vi "Example_SingleSquare.vi"() -> ()   [LabVIEW 2019, in "VGA.lvlib"]
doc: "Use this VI to test Monitor pixel-perfect. 0= top left pixel, 307199 = bottom right pixel."
uses:
  VGA.lvlib
  <vilib>/Platform/TimedLoop/XDataNode/timing_clust.ctl
  <vilib>/Platform/TimedLoop/XDataNode/nitl_modes.ctl
  <vilib>/Platform/TimedLoop/XDataNode/wakeup.ctl
  <vilib>/rvi/Emulation/niFpgaGetClockAttributes.vi
  <vilib>/rvi/Emulation/niFpgaSctlEmulationGetInTimedLoop.vi
  <vilib>/rvi/Emulation/niFpgaEmulationReportErrorSimple.vi
  <vilib>/rvi/Emulation/niFpgaCriticalErrorInLSC.vi
  <vilib>/rvi/Memory/Memory_Emulation/nirvimemoryFastEmulation.vi
  <vilib>/rvi/Memory/Memory_Emulation/nirvimemoryEmulation.vi
  <vilib>/rvi/Emulation/niFpgaEmulationIsFPGAContextNoSignature.vi
  <vilib>/rvi/DataTransferAndStorage/Container/Common/niFpgaContainerGetUniqueNameForEmu.vi
  <vilib>/rvi/Emulation/niFpgaProcessEmulError.vi
  <vilib>/rvi/errors/nirviReportUnexpectedCaseInternalError (U32).vi
  <vilib>/platform/TimedLoop/XDataNode/XDataNode.xnode
  <vilib>/rvi/DataTransferAndStorage/Container/XNode/niFpgaContainer.xnode
  <vilib>/Platform/TimedLoop/XDataNode/XDNodeRunTimeDep.lvlib
panel:
  in  "Background Color":fxp<+,3,3>
  in  "Color":fxp<+,3,3>
  in  "Height":u16
  in  "PosY":u16
  in  "Width":u16
  in  "PosX":u16
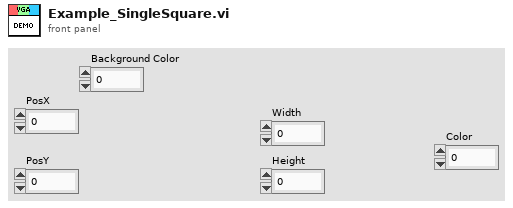
[diagram p1: front panel]
types:
  T1 = typedef "XDNodeRunTimeDep.lvlib/timing_clust.ctl" = cluster{"Expected End [f-1]":u64, "Actual End [f-1]":u64, "Finished Late? [f-1]":bool, "Expected End [i-1]":u64, "Actual End [i-1]":u64, "Finished Late? [i-1]":bool, "Expected Start [i]":u64, "Actual Start [i]":u64, "Expected Start [f]":u64, "Actual Start [f]":u64, "Source Name":string, "Structure Name":string, "Period":i64, "Deadline":i64, "Offset":i64, "Start":i64, "Priority":i32, "Timeout":i32, "Mode":T2, "Wakeup Reason":T3, "Error":errorcluster, "Source Type":string, "Secondary Source Type":string, "Global End Time":u64, "Global Start Time":u64, "Frame Duration":u64, "Iteration Duration":u64, "Assigned CPU":i32, "I/O Scan Engine Mode":u32}
  T2 = typedef "XDNodeRunTimeDep.lvlib/nitl_modes.ctl" = enum32{"No Change", "Process missed periods, maintain original phase", "Discard missed periods, maintain original phase", "Process missed periods, ignore original phase", "Discard missed periods, ignore original phase"}
  T3 = typedef "XDNodeRunTimeDep.lvlib/wakeup.ctl" = enum32{"Normal", "Aborted", "Asynchronous wakeup", "Timing source error", "Timed loop error", "Timeout"}
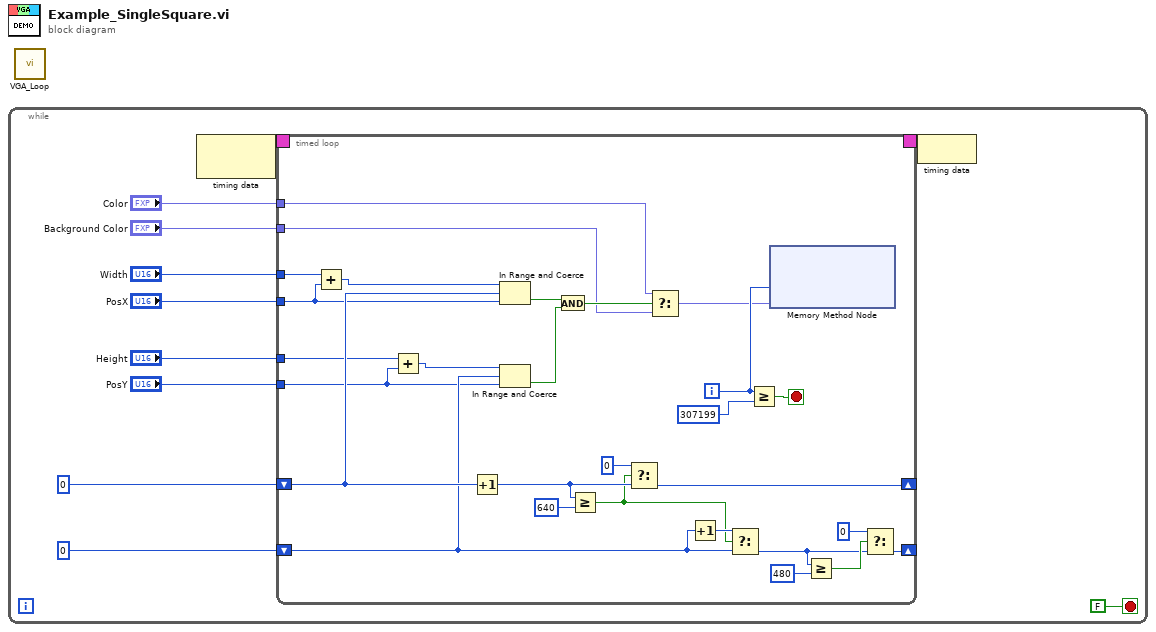
[diagram p0: block diagram]
diagram:
  n1 = while {
    stop <- FALSE stop-if-true
    n2 = node-c288() -> (w10:T1)  [unwired: 1 in]
    n3 = timed-loop {
      timing: w10 -> [_]
      timing-out: [_] -> w9
      tunnel: "PosX" -> [w24]
      shift-right: [w36] -> _
      shift-left: u16 0 ("Width") -> [w25]
      shift-right: [w29] -> _
      shift-left: u16 0 ("Width") -> [w21]
      tunnel: "Width" -> [w23]
      tunnel: "PosY" -> [w20]
      tunnel: "Height" -> [w19]
      tunnel: "Color" -> [w14]
      tunnel: "Background Color" -> [w13]
      i -> [w39]
      stop <- w38 stop-if-true
      n4 = Add(x=w23, y=w24) -> (x+y=w22:u16)
      n5 = Add(x=w19, y=w20) -> (x+y=w18:u16)
      n6 = Increment(x=w25) -> (x+1=w35:u16)
      n7 = In Range and Coerce(upper limit=w22, x=w25, lower limit=w24) -> (In Range?=w17:bool)  [unwired: 1 out]
      n8 = In Range and Coerce(upper limit=w18, x=w21, lower limit=w20) -> (In Range?=w16:bool)  [unwired: 1 out]
      n9 = And(x=w17, y=w16) -> (x .and. y?=w15:bool)
      n10 = Greater Or Equal?(x=w35, y=u16 640) -> (x >= y?=w26:bool)
      n11 = Select(t=u16 0, s=w26, f=w35) -> (s? t:f=w36:u16)
      n12 = Select(t=w14, s=w15, f=w13) -> (s? t:f=w12:fxp<+,3,3>)
      n13 = Increment(x=w21) -> (x+1=w30:u16)
      n14 = Select(t=w30, s=w26, f=w21) -> (s? t:f=w27:u16)
      n15 = Greater Or Equal?(x=w39, y=307199) -> (x >= y?=w38:bool)
      n16 = xnode ("Memory Method Node")("Address"=w39, "Data"=w12) -> ()  [unwired: 1 in, 1 out]
      n17 = Greater Or Equal?(x=w27, y=u16 480) -> (x >= y?=w31:bool)
      n18 = Select(t=u16 0, s=w31, f=w27) -> (s? t:f=w29:u16)
    }
    n19 = node-c288(w9) -> ()
  }
  n20 = call "VGA_Loop.vi"() -> ()  [unwired: 12 in]
